vi "Common Cases.vi"(8 "error in":errorcluster, 11 "Comm Worker in":refnum<class "Comm Worker.lvclass">) -> (0 "error out":errorcluster, 3 "Comm Worker out":refnum<class "Comm Worker.lvclass">)   [LabVIEW 2018, in "Comm Worker.lvclass"]
uses:
  Comm Worker.lvclass
  D:/Program Files (x86)/National Instruments/LabVIEW 2018/vi.lib/addons/_Workers/Library/Classes/Worker/Worker.lvclass
  <vilib>/addons/_Workers/Library/Classes/Worker/Worker.lvclass/Worker.ctl
  <vilib>/addons/_Workers/Library/Classes/Message/Message.lvclass/Message.ctl
  <vilib>/addons/_Workers/Library/Classes/Worker/Worker.lvclass
  <vilib>/addons/_Workers/Library/Classes/Message/Message.lvclass
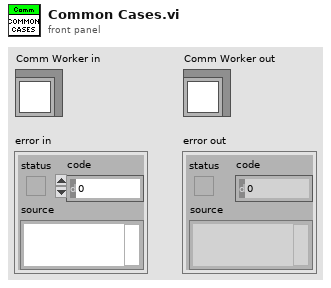
[diagram p1: front panel]
types:
  T1 = typedef "Workers.lvlib/Case Label.ctl" = string
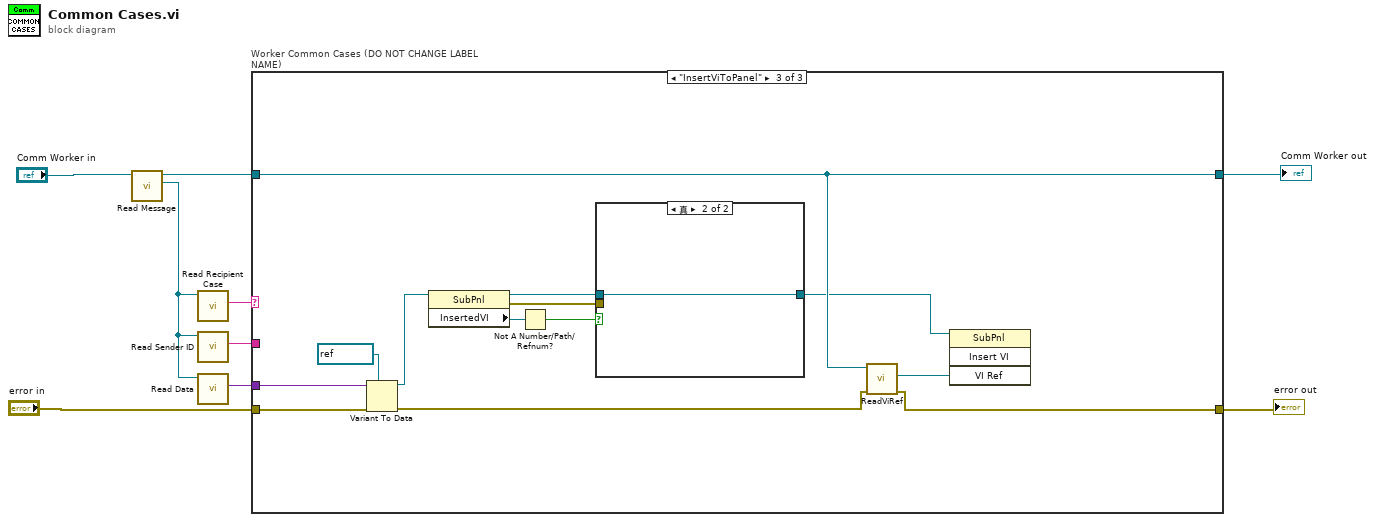
[diagram p0: block diagram]
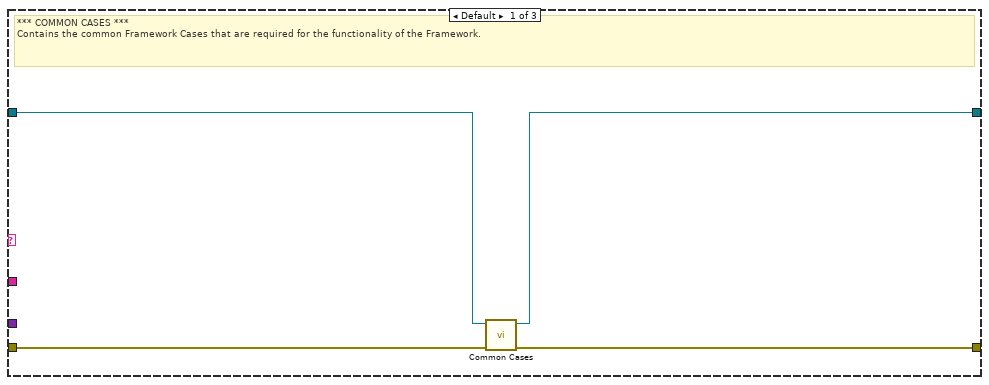
[diagram p2: hidden frame]
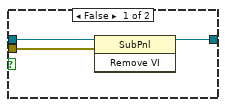
[diagram p4: hidden frame]
diagram:
  n1 = call <vilib>:"Read Message.vi"("Worker"="Comm Worker in") -> ("Message"=w6:refnum<class "Message.lvclass">, "dup Worker out"=w9:refnum<class "Comm Worker.lvclass">)  [unwired: 9 in]
  n2 = call <vilib>:"Read Recipient Case.vi"("Message"=w6) -> ("Recipient Case"=w7:T1)  [unwired: 9 in, 1 out]
  n3 = call <vilib>:"Read Sender ID.vi"("Message"=w6) -> ("Sender ID"=w5:string)  [unwired: 9 in, 1 out]
  n4 = call <vilib>:"Read Data.vi"("Message"=w6) -> ("Data"=w8:variant)  [unwired: 9 in, 1 out]
  n5 = case "Worker Common Cases (DO NOT CHANGE LABEL NAME)" shown="\"InsertViToPanel\"" w7 {
    tunnel: [w13 w15 w22] -> w2
    tunnel: [w12 w14 w25] -> w1
    tunnel: "error in" -> [w11 w15 w26]
    tunnel: w9 -> [w10 w14 w25]
    tunnel: w8 -> [_ _ w27]
    tunnel: w5 -> [_ _ _]
    frame Default {
      # "*** COMMON CASES ***\nContains the common Framework Cases that are required for the functionality of the Framework."
      n6 = call-parent "Common Cases.vi"("error in"=w11, "Worker in"=w10) -> ("error out"=w13:errorcluster, "Worker out"=w12:refnum<class "Comm Worker.lvclass">)  [unwired: 8 in]
    }
    frame "-------CommMessage------" {
    }
    frame "InsertViToPanel" {
      n7 = Variant To Data(error in=w26, type=refnum<vi> refnum ("子面板"), Variant=w27) -> (data=w17:refnum<vi>, error out=w23:errorcluster)
      n8 = property class="SubPnl"(reference=w17) -> (reference out=w20:refnum<vi>, error out=w19:errorcluster, "InsertedVI"=w21:refnum<vi>)  [unwired: 1 in]
      n9 = Not A Number/Path/Refnum?(number/path/refnum=w21) -> (NaN/Path/Refnum?=w18:bool)
      n10 = case shown="真" w18 {
        tunnel: w20 -> [w31 w32]
        tunnel: w19 -> [w30 _]
        tunnel: [w29 w32] -> w16
        frame False {
          n11 = invoke class="SubPnl" method="Remove VI"(reference=w31, error in=w30) -> (reference out=w29:refnum<vi>)  [unwired: 1 in, 2 out]
        }
        frame True {
        }
      }
      n12 = call-dynamic "ReadViRef.vi"("error in (no error)"=w23, "Comm Worker 输入"=w25) -> ("error out"=w22:errorcluster, "VI"=w24:refnum<vi>)  [unwired: 7 in, 1 out]
      n13 = invoke class="SubPnl" method="Insert VI"(reference=w16, "VI Ref"=w24) -> ()  [unwired: 2 in, 4 out]
    }
  }
  "Comm Worker out" <- w1
  "error out" <- w2
